vi "Write dc.vi"(8 "error in (no error)":errorcluster, 10 "dc":dbl, 11 "Heater Data in":refnum<class "Heater Data.lvclass">) -> (0 "error out":errorcluster, 3 "Heater Data out":refnum<class "Heater Data.lvclass">)   [LabVIEW 2017, in "Controller.lvlib" / "Heater Data.lvclass"]
uses:
  Heater Data.lvclass
  Heater Data.lvclass/Heater Data.ctl
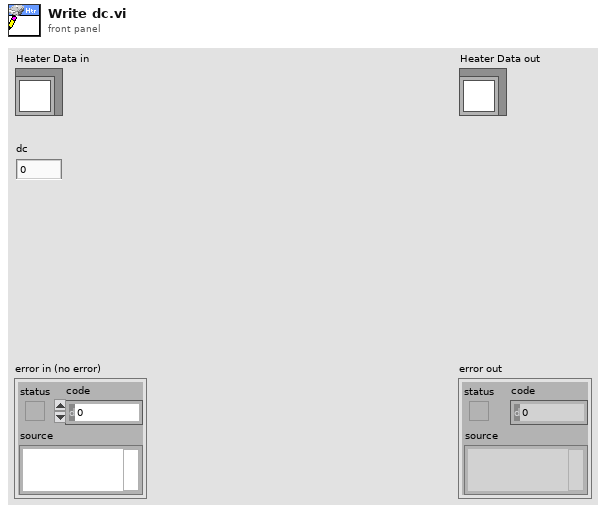
[diagram p1: front panel]
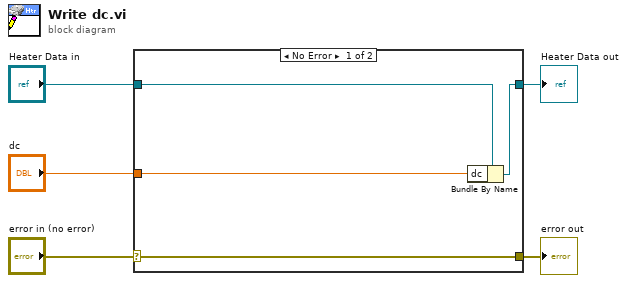
[diagram p0: block diagram]
diagram:
  n1 = case shown="No Error" "error in (no error)" {
    selector: "error in (no error)" -> [w9 w10]
    tunnel: [w9 w10] -> w4
    tunnel: [w7 w11] -> w2
    tunnel: "Heater Data in" -> [w8 w11]
    tunnel: "dc" -> [w6 _]
    frame No Error {
      n2 = Bundle By Name(cluster=w8, "dc"=w6) -> (w7:refnum<class "Heater Data.lvclass">)
    }
    frame Error {
    }
  }
  "error out" <- w4
  "Heater Data out" <- w2
